vi "ManualControlL0.vi"() -> ()   [LabVIEW 2012]
uses:
  <vilib>/Utility/NIReport.llb/NI_report.lvclass
  <vilib>/Utility/NIReport.llb/HTML/NI_HTML.lvclass
panel:
  in  "Amp Scaler":dbl(slide)=0.1 scale=0.1..10.0
  in  "Voltage Input":dbl(slide)=0.5015306122448979 scale=0.05..0.8
  in  "Sum/Maj":bool=TRUE
  in  "Ib Clip select":i32(slide)=63 scale=0.0..63.0
  in  "Clipping Select":i32(slide)=1 scale=1.0..3.0
  in  "Attenuation Select":i32(slide) scale=0.0..15.0
  in  "Delay Enable":i32(slide) scale=0.0..31.0
  in  "Channel Enable":i32(slide) scale=0.0..6.0
  in  "stop":bool
  in  "Instrument VISA in":T1={"AWG VISA"="AgilentGenerator1", "Oscilloscope  VISA "="AgilentOsciloscope", "Integration Board IP"="172.16.17.47", "connection ID"=refnum, "report out"=refnum, "report file path"=path "C:/Documents and Settings/CTA_LAB01/Desktop/L0_Asic/L0 Asic Test Data"}
  out "error out":errorcluster
  in  "error in (no error)":errorcluster
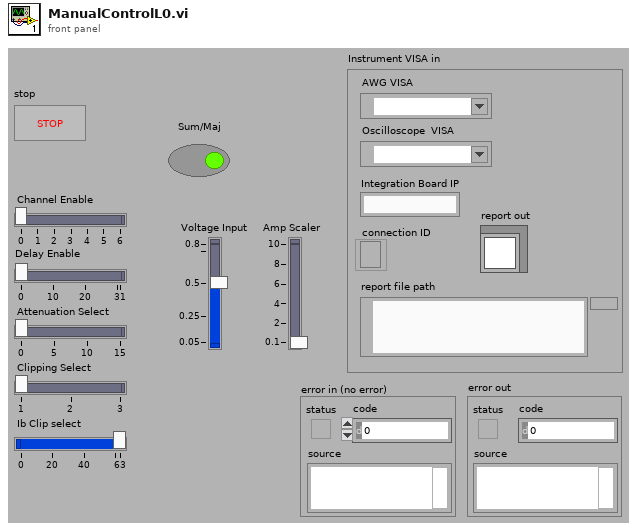
[diagram p1: front panel]
types:
  T1 = cluster{"AWG VISA":refnum<visa-resource-name>, "Oscilloscope  VISA ":refnum<visa-resource-name>, "Integration Board IP":string, "connection ID":refnum<k5>, "report out":refnum<class "NI_report.lvclass">, "report file path":path}
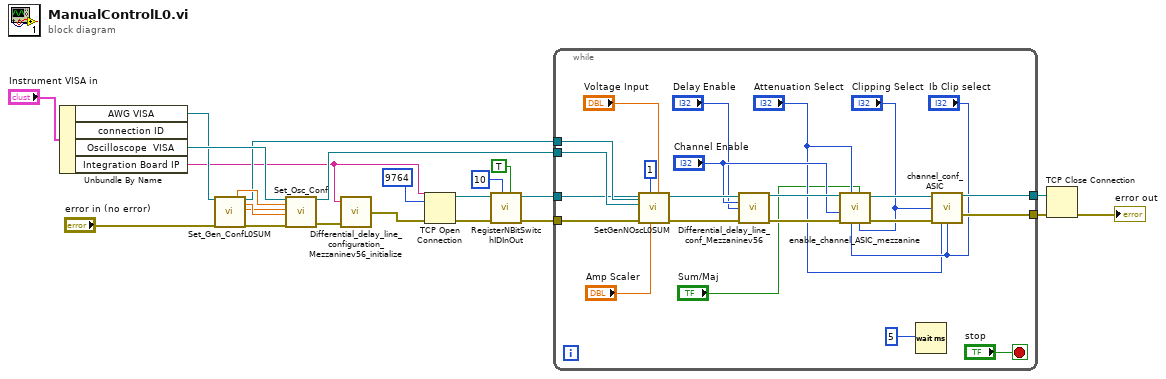
[diagram p0: block diagram]
diagram:
  n1 = Unbundle By Name("Instrument VISA in") -> ("AWG VISA"=w18:refnum<visa-resource-name>, "Oscilloscope  VISA"=w19:refnum<visa-resource-name>, "Integration Board IP"=w1:string)  [unwired: 1 out]
  n2 = call "Set_Gen_ConfL0SUM.vi"("AWG VISA"=w18, "error in (no error)"="error in (no error)") -> ("Amplitude 1 OUT"=w16:dbl, "VISA resource name out"=w7:refnum<visa-resource-name>, "Pulse Width in seconds 1 OUT"=w15:dbl, "Trigger Level 1"=w14:dbl, "error out"=w21:errorcluster)  [unwired: 10 in, 3 out]
  n3 = call "Set_Osc_Conf.vi"("VISA resource name"=w19, "Amplitude IN"=w16, "Trigger Level IN"=w14, "Pulse Width in seconds IN"=w15, "error in (no error)"=w21) -> ("VISA resource name out"=w8:refnum<visa-resource-name>, "error out"=w13:errorcluster)  [unwired: 13 in]
  n4 = call "Differential_delay_line_configuration_Mezzaninev56_initialize.vi"("error in (no error)"=w13, "address"=w1) -> ("error out 2"=w12:errorcluster)  [unwired: 1 in]
  n5 = TCP Open Connection(address=w1, remote port or service name=9764, error in (no error)=w12) -> (connection ID=w5:refnum<k5>, error out=w11:errorcluster)  [unwired: 2 in]
  n6 = call "RegisterNBitSwitchIDInOut.vi"("Switch Bit"=TRUE, "N Bit"=10, "error in (no error)"=w11, "connection ID"=w5) -> ("error out"=w6:errorcluster, "connection ID out"=w4:refnum<k5>)  [unwired: 5 in]
  n7 = while {
    tunnel: [w45] -> w10
    tunnel: [w44] -> w9
    tunnel: w8 -> [w43]
    tunnel: w7 -> [w42]
    tunnel: w6 -> [w41]
    tunnel: w4 -> [w40]
    stop <- "stop" stop-if-true
    n8 = call "SetGenNOscL0SUM.vi"("Input Voltage"="Voltage Input", "Amp Scaler"="Amp Scaler", "NChannels"=1, "error in (no error)"=w41, "VISA resource name"=w43, "AWG VISA"=w42) -> ("error out 2"=w39:errorcluster)  [unwired: 5 in]
    n9 = call "Differential_delay_line_conf_Mezzaninev56.vi"("connection ID"=w40, "channel"="Channel Enable", "Delay value"="Delay Enable", "error in (no error)"=w39) -> ("connection ID out"=w33:refnum<k5>, "error out 2"=w35:errorcluster)  [unwired: 4 in, 6 out]
    n10 = call "enable_channel_ASIC_mezzanine.vi"("Clip_sel_b"="Clipping Select", "maj/sum"="Sum/Maj", "Ib_clipVb"="Ib Clip select", "Att gain"="Attenuation Select", "error in"=w35, "Channel"="Channel Enable", "connection ID"=w33) -> ("error out"=w34:errorcluster, "connection ID out"=w32:refnum<k5>)  [unwired: 2 in, 1 out]
    n11 = Wait (ms)(milliseconds to wait=5) -> ()  [unwired: 1 out]
    n12 = call "channel_conf_ASIC.vi"("connection ID"=w32, "Clip_sel_b"="Clipping Select", "error out"=w34, "Att gain"="Attenuation Select", "Ib_ClipVb"="Ib Clip select") -> ("connection ID out"=w44:refnum<k5>, "error out 2"=w45:errorcluster)  [unwired: 6 in, 3 out]
  }
  n13 = TCP Close Connection(connection ID=w9, error in (no error)=w10) -> (error out=→"error out":errorcluster)  [unwired: 1 in, 1 out]
